vi "ConfigHelper.vi"(0 "object in":refnum<class "MTEC_Async.lvclass">, 2 "Config Data":T4={"meTEC_CH1_Input Selection (ID 2000)"=2, "meTEC_CH2_Input Selection (ID 2000)"=2, "meTEC_CH1_Object Target Temp. Source Selection (ID 50011)"=0, "meTEC_CH2_Object Target Temp. Source Selection (ID 50011)"=0, "meTEC_CH1_Live Enable (ID 50000)"=0, "meTEC_CH2_Live Enable (ID 50000)"=0, "meTEC_CH1_Object Target Temperature (ID 3000 / 50012) [°C]"=23.0, "meTEC_CH2_Object Target Temperature (ID 3000 / 50012) [°C]"=23.0, "meTEC_CH1_Live Set Current (ID 50001) [A]"=0.0, "meTEC_CH2_Live Set Current (ID 50001) [A]"=0.0, "meTEC_CH1_Live Set Voltage (ID 50002) [V]"=0.0, "meTEC_CH2_Live Set Voltage (ID 50002) [V]"=0.0} {"meTEC_CH2_Live Set Voltage (ID 50002) [V]" min=0.0 max=22.000001907348633 step=0.001 format="%#.3f"; "meTEC_CH1_Live Set Voltage (ID 50002) [V]" min=0.0 max=0.0 step=0.001 format="%#.3f"; "meTEC_CH2_Live Set Current (ID 50001) [A]" min=-10.0 max=10.0 step=0.001 format="%#.3f"; "meTEC_CH1_Live Set Current (ID 50001) [A]" min=0.0 max=0.0 step=0.001 format="%#.3f"; "meTEC_CH2_Object Target Temperature (ID 3000 / 50012) [°C]" min=-273.0 max=1000.0 step=0.001 format="%#.3f"; "meTEC_CH1_Object Target Temperature (ID 3000 / 50012) [°C]" min=0.0 max=0.0 step=0.001 format="%#.3f"; "meTEC_CH2_Live Enable (ID 50000)" items=["Disabled (Reset State)", "Enabled"]; "meTEC_CH1_Live Enable (ID 50000)" items=["Disabled (Reset State)", "Enabled"]; "meTEC_CH2_Object Target Temp. Source Selection (ID 50011)" items=["Parameter ID 3000 (Reset State)", "Parameter ID 50012"]; "meTEC_CH1_Object Target Temp. Source Selection (ID 50011)" items=["Parameter ID 3000 (Reset State)", "Parameter ID 50012"]; "meTEC_CH2_Input Selection (ID 2000)" items=["Static Current / Voltage", "Live Current / Voltage", "Temperature Controller"]; "meTEC_CH1_Input Selection (ID 2000)" items=["Static Current / Voltage", "Live Current / Voltage", "Temperature Controller"]}, 5 "error in (no error)":errorcluster) -> (14 "object out":refnum<class "MTEC_Async.lvclass">, 19 "error out":errorcluster)   [LabVIEW 2019, in "MTEC_Async.lvclass"]
uses:
  MTEC_Async.lvclass
  TEC LabVIEW Control Software v0.14/Source/LV Source/[meerstetter engineering TE Cooling]/TypeDefs/meTEC_ID 2000_Input Selection.ctl
  TEC LabVIEW Control Software v0.14/Source/LV Source/[meerstetter engineering TE Cooling]/TypeDefs/meTEC_ID 50011_Object Target Temperature Source Selection.ctl
  TEC LabVIEW Control Software v0.14/Source/LV Source/[meerstetter engineering TE Cooling]/TypeDefs/meTEC_ID 50000_Live Enable.ctl
  MTEC_Async.lvclass/MTEC_Async.ctl
  TEC LabVIEW Control Software v0.14/Source/LV Source/Variables/FGVs/Type Defs/FGV_Operations.ctl
panel:
  in  "meTEC_CH2_Live Set Voltage (ID 50002) [V]":dbl caption="Live Set Voltage (ID 50002) [V]" min=0.0 max=22.000001907348633 step=0.001 format="%#.3f"
  in  "meTEC_CH1_Live Set Voltage (ID 50002) [V]":dbl caption="Live Set Voltage (ID 50002) [V]" min=0.0 max=0.0 step=0.001 format="%#.3f"
  in  "meTEC_CH2_Live Set Current (ID 50001) [A]":dbl caption="Live Set Current (ID 50001) [A]" min=-10.0 max=10.0 step=0.001 format="%#.3f"
  in  "meTEC_CH1_Live Set Current (ID 50001) [A]":dbl caption="Live Set Current (ID 50001) [A]" min=0.0 max=0.0 step=0.001 format="%#.3f"
  in  "meTEC_CH2_Object Target Temperature (ID 3000 / 50012) [°C]":dbl
  in  "meTEC_CH1_Object Target Temperature (ID 3000 / 50012) [°C]":dbl=23.0 caption="Object Target Temperature (ID 3000 / 50012) [°C]" min=0.0 max=0.0 step=0.001 format="%#.3f"
  in  "meTEC_CH2_Live Enable (ID 50000)":T1 caption="Live Enable" items=["Disabled (Reset State)", "Enabled"]
  in  "meTEC_CH1_Live Enable (ID 50000)":T1 caption="Live Enable (ID 50000)" items=["Disabled (Reset State)", "Enabled"]
  in  "meTEC_CH2_Object Target Temp. Source Selection (ID 50011)":T2 caption="Object Target Temperature Source Selection (ID 50011)" items=["Parameter ID 3000 (Reset State)", "Parameter ID 50012"]
  in  "meTEC_CH1_Object Target Temp. Source Selection (ID 50011)":T2 caption="Object Target Temperature Source Selection (ID 50011)" items=["Parameter ID 3000 (Reset State)", "Parameter ID 50012"]
  in  "meTEC_CH2_Input Selection (ID 2000)":T3=2 caption="Input  Selection (ID 2000)" items=["Static Current / Voltage", "Live Current / Voltage", "Temperature Controller"]
  in  "meTEC_CH1_Input Selection (ID 2000)":T3=2 caption="Input  Selection (ID 2000)" items=["Static Current / Voltage", "Live Current / Voltage", "Temperature Controller"]
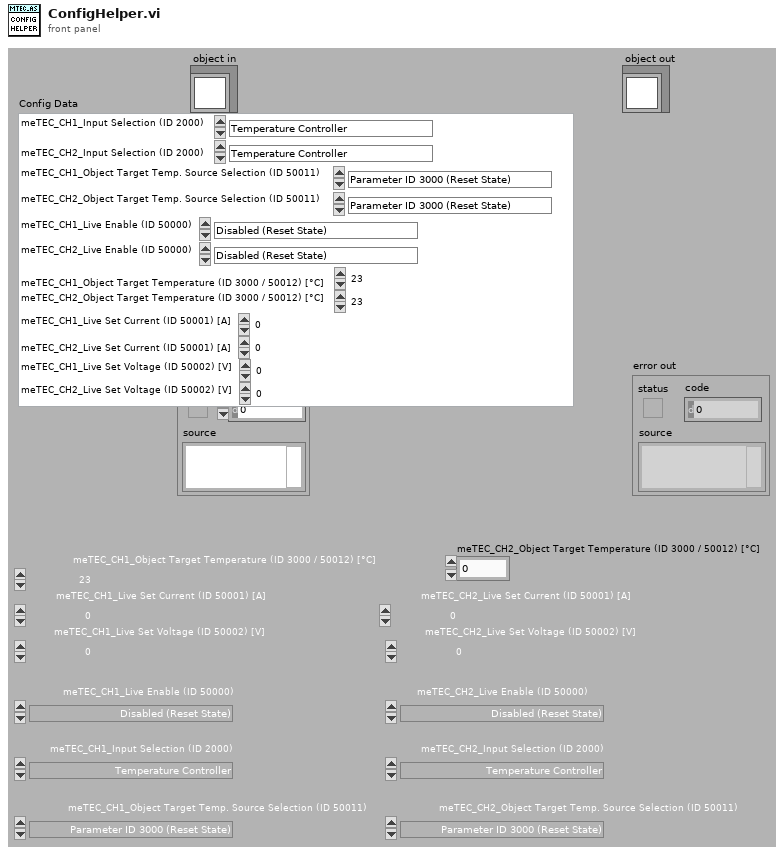
[diagram p1: front panel]
types:
  T1 = typedef "meTEC_ID 50000_Live Enable.ctl" = i32
  T2 = typedef "meTEC_ID 50011_Object Target Temperature Source Selection.ctl" = i32
  T3 = typedef "meTEC_ID 2000_Input Selection.ctl" = i32
  T4 = cluster{"meTEC_CH1_Input Selection (ID 2000)":T3, "meTEC_CH2_Input Selection (ID 2000)":T3, "meTEC_CH1_Object Target Temp. Source Selection (ID 50011)":T2, "meTEC_CH2_Object Target Temp. Source Selection (ID 50011)":T2, "meTEC_CH1_Live Enable (ID 50000)":T1, "meTEC_CH2_Live Enable (ID 50000)":T1, "meTEC_CH1_Object Target Temperature (ID 3000 / 50012) [°C]":dbl, "meTEC_CH2_Object Target Temperature (ID 3000 / 50012) [°C]":dbl, "meTEC_CH1_Live Set Current (ID 50001) [A]":dbl, "meTEC_CH2_Live Set Current (ID 50001) [A]":dbl, "meTEC_CH1_Live Set Voltage (ID 50002) [V]":dbl, "meTEC_CH2_Live Set Voltage (ID 50002) [V]":dbl}
  T5 = typedef "FGV_Operations.ctl" = enum16{"Read", "Write"}
  T6 = typedef "FGV_TE Controller.ctl" = cluster{"SVs":cluster{"Unused":dbl}, "PVs":cluster{"FW & HW Versions":cluster{"Device Type [I32]":i32, "Device Type [String]":string, "Firmware Version [I32]":i32, "Firmware Version [String]":string, "Hardware Version [I32]":i32, "Hardware Version [String]":string, "Serial No.":i32}, "TEC Configuration":T7, "Object Target Temperature Source_CH1":u8, "Object Target Temperature Source_CH2":u8}, "Front Panel References":T8}
  T7 = typedef "meTEC_Configuration.ctl" = cluster{"VISA resource name":refnum<visa-resource-name>, "Device Address":u16}
  T8 = typedef "FGV_Front Panel References.ctl" = cluster{"Main Loop Queue":refnum<queue>, "meTEC_Device Type":refnum<vi>, "meTEC_Serial No.":refnum<vi>, "meTEC_Hardware Version":refnum<vi>, "meTEC_Firmware Version":refnum<vi>, "meTEC_CH1_Object Target Temperature (ID 3000 / 50012) [°C]":refnum<vi>, "meTEC_CH1_Live Set Current (ID 50001) [A]":refnum<vi>, "meTEC_CH1_Live Set Voltage (ID 50002) [V]":refnum<vi>, "meTEC_CH1_Live Enable (ID 50000)":refnum<vi>, "meTEC_CH1_Input Selection (ID 2000)":refnum<vi>, "meTEC_CH1_Object Target Temp. Source Sel. (ID 50011)":refnum<vi>, "meTEC_CH2_Object Target Temperature (ID 3000 / 50012) [°C]":refnum<vi>, "meTEC_CH2_Live Set Current (ID 50001) [A]":refnum<vi>, "meTEC_CH2_Live Set Voltage (ID 50002) [V]":refnum<vi>, "meTEC_CH2_Live Enable (ID 50000)":refnum<vi>, "meTEC_CH2_Input Selection (ID 2000)":refnum<vi>, "meTEC_CH2_Object Target Temp. Source Sel. (ID 50011)":refnum<vi>, "meTEC_CH2_Object Temperature [°C]":refnum<vi>, "meTEC_CH2_Sink Temperature [°C]":refnum<vi>, "meTEC_CH2_Act. Output Current [A]":refnum<vi>, "meTEC_CH2_Act. Output Voltage [V]":refnum<vi>, "meTEC_CH2_Temperature Stability":refnum<vi>, "Monitor Chart_CH2":refnum<vi>, "meTEC_Initialize Device":refnum<vi>}
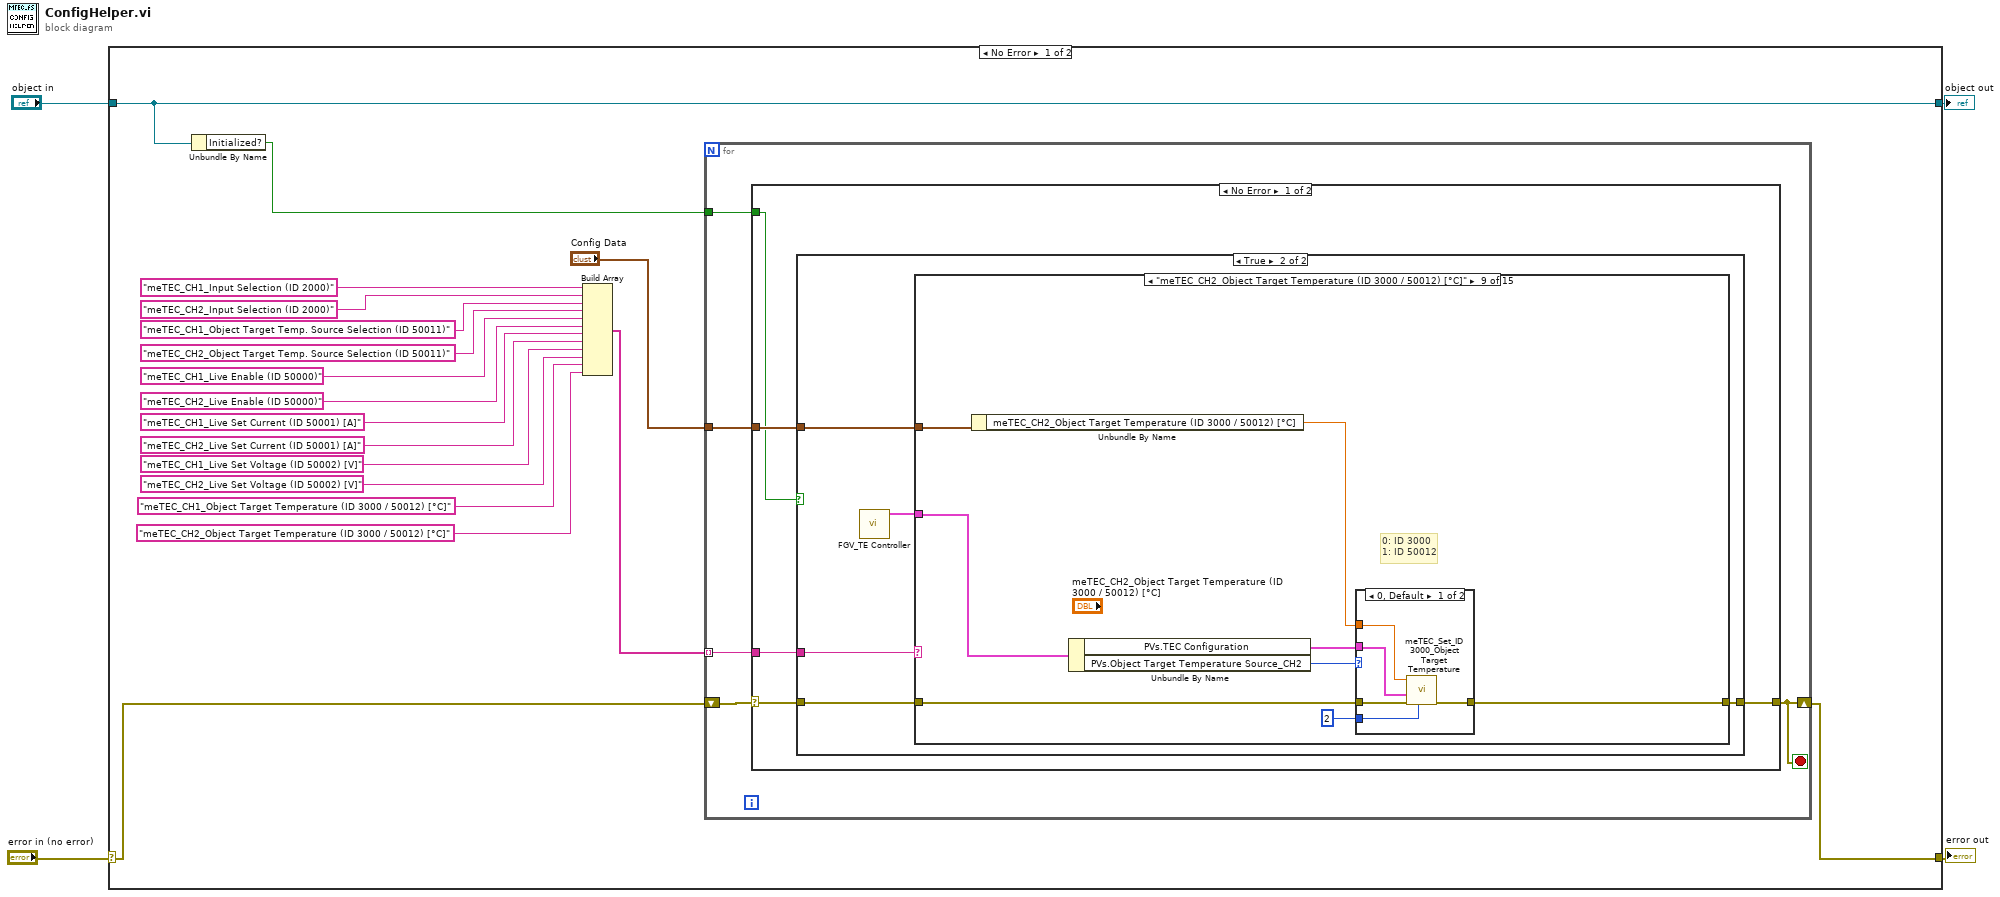
[diagram p0: block diagram]
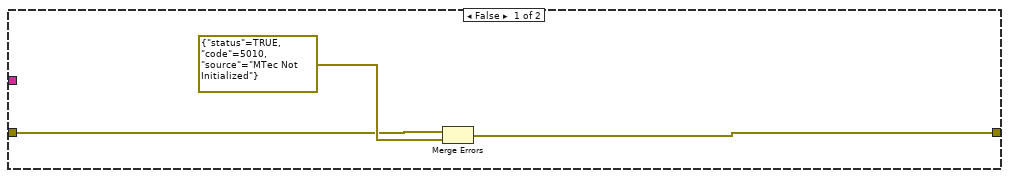
[diagram p2: hidden frame]
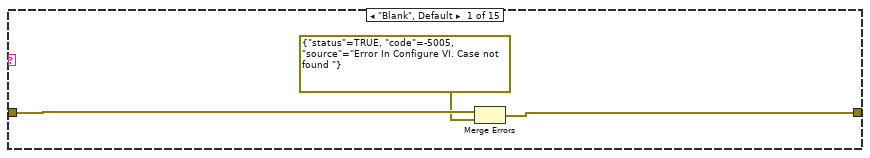
[diagram p3: hidden frame]
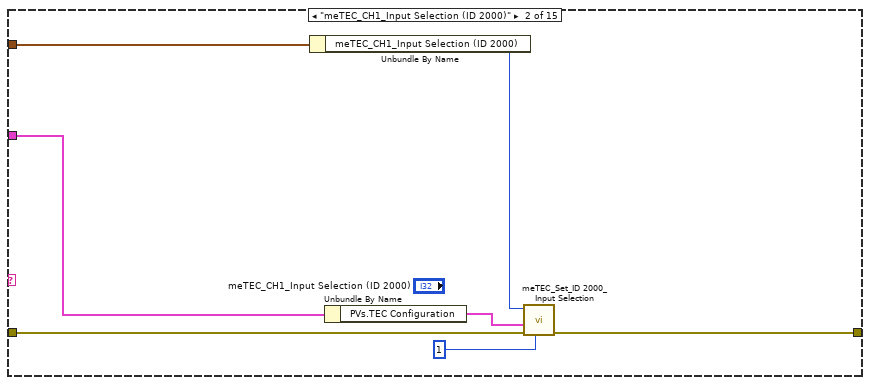
[diagram p4: hidden frame]
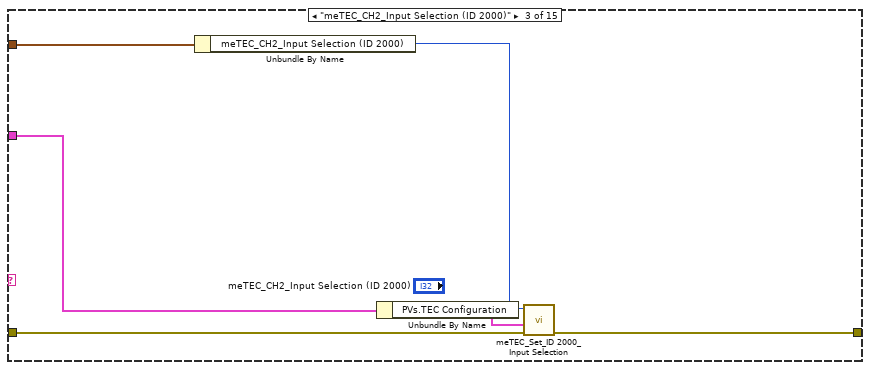
[diagram p5: hidden frame]
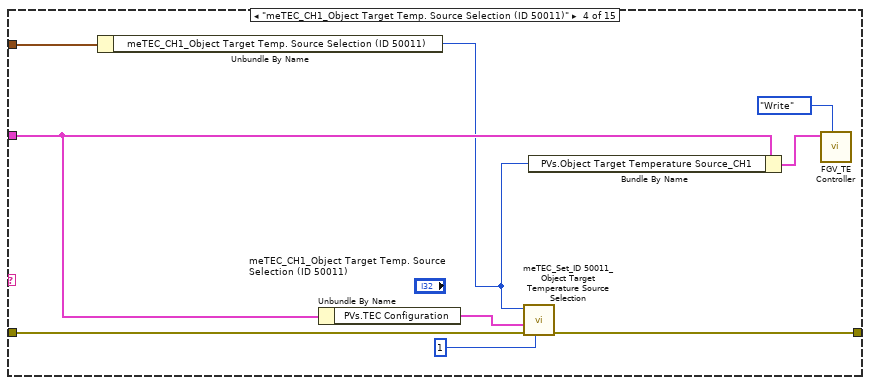
[diagram p6: hidden frame]
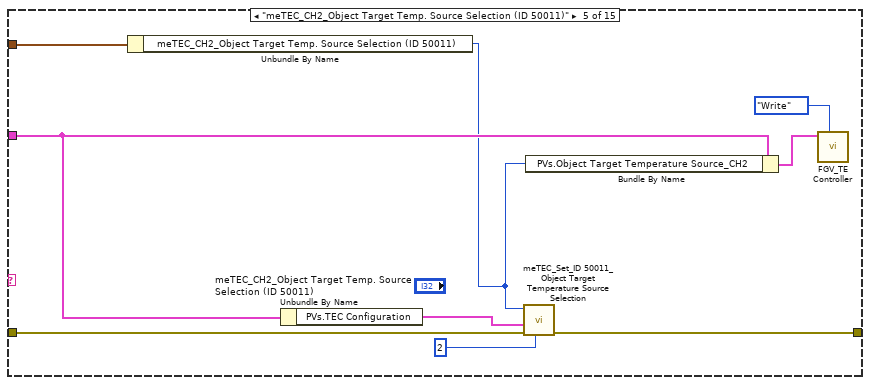
[diagram p7: hidden frame]
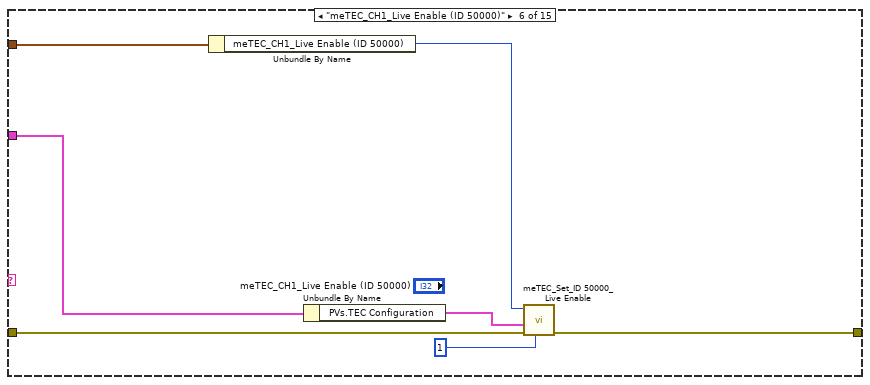
[diagram p8: hidden frame]
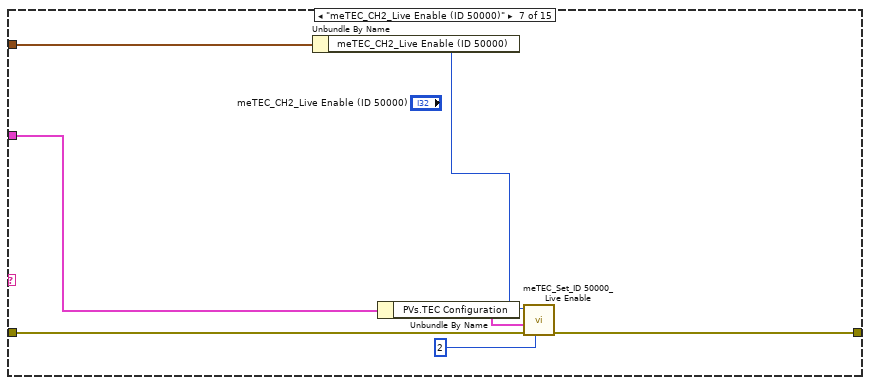
[diagram p9: hidden frame]
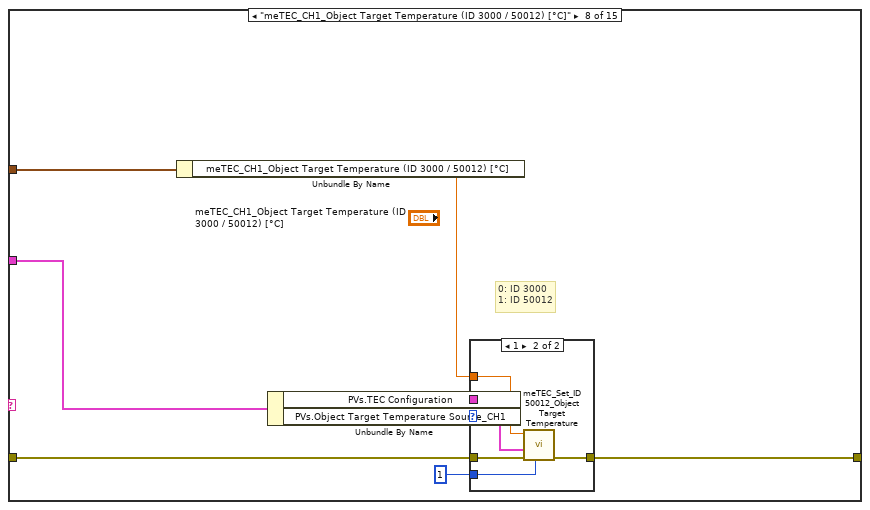
[diagram p10: hidden frame]
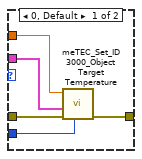
[diagram p11: hidden frame]
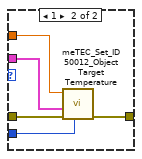
[diagram p12: hidden frame]
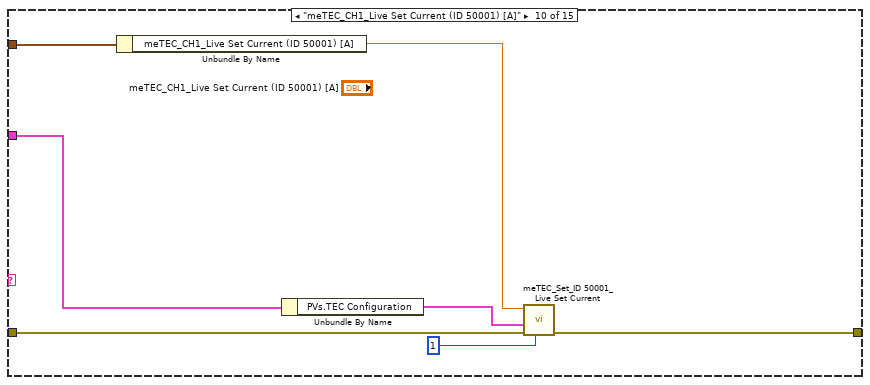
[diagram p13: hidden frame]
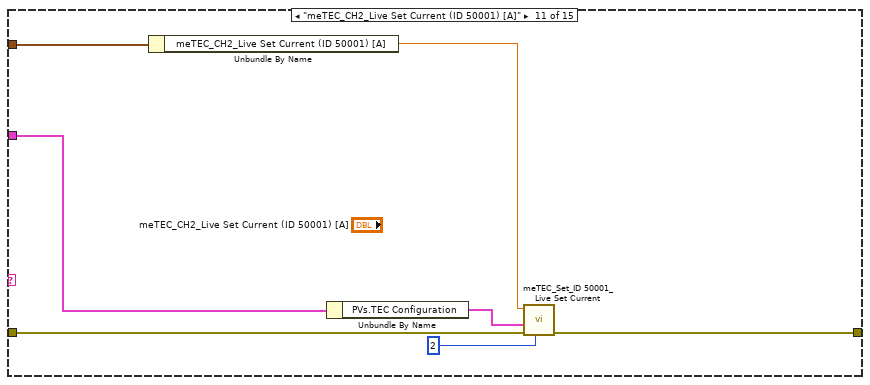
[diagram p14: hidden frame]
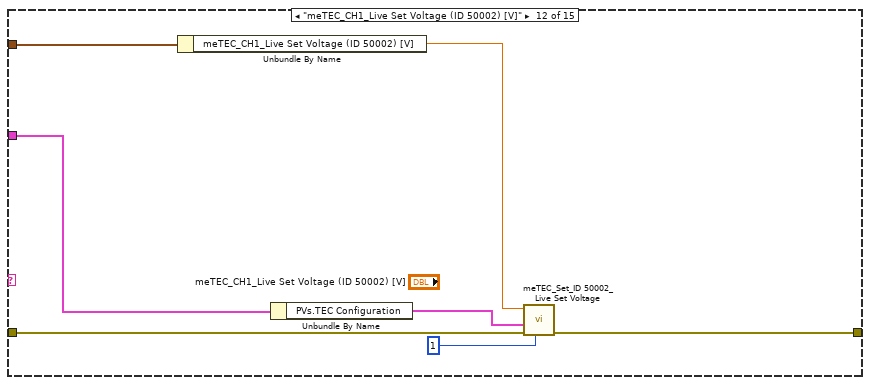
[diagram p15: hidden frame]
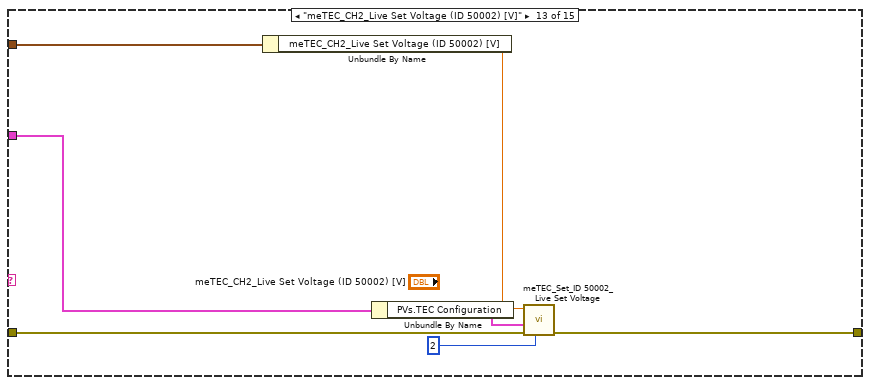
[diagram p16: hidden frame]
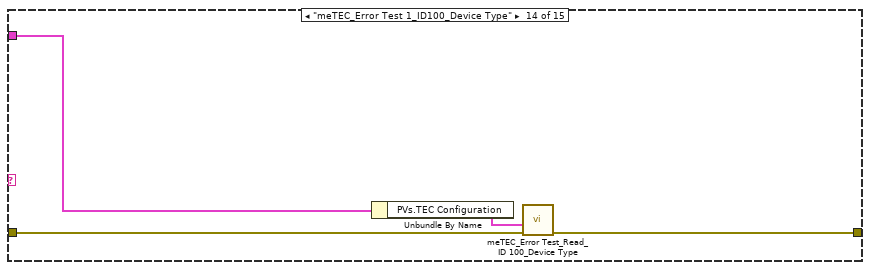
[diagram p17: hidden frame]
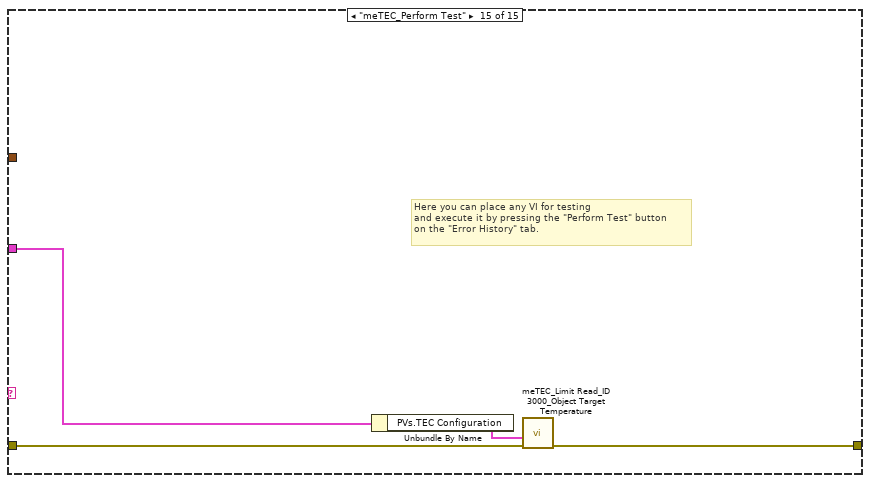
[diagram p18: hidden frame]
diagram:
  n1 = case shown="No Error" "error in (no error)" {
    selector: "error in (no error)" -> [w5 w163]
    tunnel: [w6 w163] -> w3
    tunnel: [w22 w162] -> w1
    tunnel: "object in" -> [w22 w162]
    frame No Error {
      n2 = Unbundle By Name(w22) -> ("Initialized?"=w7:bool)
      n3 = Build Array("meTEC_CH1_Input Selection (ID 2000)", "meTEC_CH2_Input Selection (ID 2000)", "meTEC_CH1_Object Target Temp. Source Selection (ID 50011)", "meTEC_CH2_Object Target Temp. Source Selection (ID 50011)", "meTEC_CH1_Live Enable (ID 50000)", "meTEC_CH2_Live Enable (ID 50000)", "meTEC_CH1_Live Set Current (ID 50001) [A]", "meTEC_CH2_Live Set Current (ID 50001) [A]", "meTEC_CH1_Live Set Voltage (ID 50002) [V]", "meTEC_CH2_Live Set Voltage (ID 50002) [V]", "meTEC_CH1_Object Target Temperature (ID 3000 / 50012) [°C]", "meTEC_CH2_Object Target Temperature (ID 3000 / 50012) [°C]") -> (w10:string[])
      n4 = for {
        tunnel: w10 -> [w26] mode=indexing
        tunnel: "Config Data" -> [w25]
        shift-right: [w23] -> w6
        shift-left: w5 -> [w27]
        tunnel: w7 -> [w24]
        stop <- w23 stop-if-true
        n5 = case shown="No Error" w27 {
          selector: w27 -> [w31 w161]
          tunnel: [w30 w161] -> w23
          tunnel: w26 -> [w32 _]
          tunnel: w25 -> [w29 _]
          tunnel: w24 -> [w28 _]
          frame No Error {
            n6 = case shown="True" w28 {
              tunnel: w32 -> [_ w39]
              tunnel: w31 -> [w33 w38]
              tunnel: [w34 w37] -> w30
              tunnel: w29 -> [_ w36]
              frame False {
                n7 = Merge Errors(w33, errorcluster {"status"=TRUE, "code"=5010, "source"="MTec Not Initialized"} ("error in (no error)")) -> (w34:errorcluster)
              }
              frame True {
                n8 = call "FGV_TE Controller.vi"() -> ("FGV_TEC_OUT"=w40:T6)  [unwired: 10 in, 1 out]
                n9 = case shown="\"meTEC_CH2_Object Target Temperature (ID 3000 / 50012) [°C]\"" w39 {
                  tunnel: w38 -> [w43 w50 w56 w65 w74 w81 w88 w96 w114 w131 w138 w145 w152 w155 w159]
                  tunnel: [w42 w49 w55 w64 w73 w80 w87 w95 w113 w130 w137 w144 w151 w153 w157] -> w37
                  tunnel: w40 -> [_ w48 w54 w61 w68 w79 w86 w94 w112 w129 w136 w143 w150 w156 w160]
                  tunnel: w36 -> [_ w45 w52 w58 w67 w76 w83 w90 w108 w126 w133 w140 w147 _ _]
                  frame "Blank", Default {
                    n10 = Merge Errors(w43, errorcluster {"status"=TRUE, "code"=-5005, "source"="Error In Configure VI. Case not found "} ("error in (no error)")) -> (w42:errorcluster)
                  }
                  frame "meTEC_CH1_Input Selection (ID 2000)" {
                    n11 = Unbundle By Name(w45) -> ("meTEC_CH1_Input Selection (ID 2000)"=w44:T3)
                    n12 = Unbundle By Name(w48) -> ("PVs.TEC Configuration"=w47:T7)
                    n13 = call "meTEC_Set_ID 2000_Input Selection.vi"("Instance (1)"=u8 1, "error in (no error)"=w50, "TEC Configuration_IN"=w47, "Input Selection (ID 2000)"=w44) -> ("error out"=w49:errorcluster)  [unwired: 5 in, 2 out]
                  }
                  frame "meTEC_CH2_Input Selection (ID 2000)" {
                    n14 = Unbundle By Name(w52) -> ("meTEC_CH2_Input Selection (ID 2000)"=w51:T3)
                    n15 = Unbundle By Name(w54) -> ("PVs.TEC Configuration"=w53:T7)
                    n16 = call "meTEC_Set_ID 2000_Input Selection.vi"("error in (no error)"=w56, "TEC Configuration_IN"=w53, "Input Selection (ID 2000)"=w51) -> ("error out"=w55:errorcluster)  [unwired: 6 in, 2 out]
                  }
                  frame "meTEC_CH1_Object Target Temp. Source Selection (ID 50011)" {
                    n17 = Unbundle By Name(w58) -> ("meTEC_CH1_Object Target Temp. Source Selection (ID 50011)"=w57:T2)
                    n18 = Unbundle By Name(w61) -> ("PVs.TEC Configuration"=w63:T7)
                    n19 = call "meTEC_Set_ID 50011_Object Target Temperature Source Selection.vi"("Instance (1)"=u8 1 ("Instance (0)"), "error in (no error)"=w65, "TEC Configuration_IN"=w63, "Object Target Temperature Source Selection (ID 50011)"=w57) -> ("error out"=w64:errorcluster)  [unwired: 5 in, 2 out]
                    n20 = Bundle By Name(cluster=w61, "PVs.Object Target Temperature Source_CH1"=w57) -> (w60:T6)
                    n21 = call "FGV_TE Controller.vi"("Operation (Read)"=FGV_Operations."Write", "FGV_TEC_IN"=w60) -> ()  [unwired: 8 in, 2 out]
                  }
                  frame "meTEC_CH2_Object Target Temp. Source Selection (ID 50011)" {
                    n22 = Unbundle By Name(w67) -> ("meTEC_CH2_Object Target Temp. Source Selection (ID 50011)"=w66:T2)
                    n23 = Unbundle By Name(w68) -> ("PVs.TEC Configuration"=w72:T7)
                    n24 = call "meTEC_Set_ID 50011_Object Target Temperature Source Selection.vi"("Instance (1)"=u8 2 ("Instance (0)"), "error in (no error)"=w74, "TEC Configuration_IN"=w72, "Object Target Temperature Source Selection (ID 50011)"=w66) -> ("error out"=w73:errorcluster)  [unwired: 5 in, 2 out]
                    n25 = Bundle By Name(cluster=w68, "PVs.Object Target Temperature Source_CH2"=w66) -> (w69:T6)
                    n26 = call "FGV_TE Controller.vi"("Operation (Read)"=FGV_Operations."Write", "FGV_TEC_IN"=w69) -> ()  [unwired: 8 in, 2 out]
                  }
                  frame "meTEC_CH1_Live Enable (ID 50000)" {
                    n27 = Unbundle By Name(w76) -> ("meTEC_CH1_Live Enable (ID 50000)"=w75:T1)
                    n28 = Unbundle By Name(w79) -> ("PVs.TEC Configuration"=w78:T7)
                    n29 = call "meTEC_Set_ID 50000_Live Enable.vi"("Instance (1)"=u8 1 ("Instance (0)"), "error in (no error)"=w81, "TEC Configuration_IN"=w78, "Live Enable (ID 50000)"=w75) -> ("error out"=w80:errorcluster)  [unwired: 5 in, 2 out]
                  }
                  frame "meTEC_CH2_Live Enable (ID 50000)" {
                    n30 = Unbundle By Name(w83) -> ("meTEC_CH2_Live Enable (ID 50000)"=w82:T1)
                    n31 = Unbundle By Name(w86) -> ("PVs.TEC Configuration"=w85:T7)
                    n32 = call "meTEC_Set_ID 50000_Live Enable.vi"("Instance (1)"=u8 2 ("Instance (0)"), "error in (no error)"=w88, "TEC Configuration_IN"=w85, "Live Enable (ID 50000)"=w82) -> ("error out"=w87:errorcluster)  [unwired: 5 in, 2 out]
                  }
                  frame "meTEC_CH1_Object Target Temperature (ID 3000 / 50012) [°C]" {
                    # "0: ID 3000\n1: ID 50012"
                    n33 = Unbundle By Name(w90) -> ("meTEC_CH1_Object Target Temperature (ID 3000 / 50012) [°C]"=w89:dbl)
                    n34 = Unbundle By Name(w94) -> ("PVs.TEC Configuration"=w93:T7, "PVs.Object Target Temperature Source_CH1"=w91:u8)
                    n35 = case shown="1" w91 {
                      tunnel: w96 -> [w101 w106]
                      tunnel: [w100 w105] -> w95
                      tunnel: w89 -> [w99 w104]
                      tunnel: w93 -> [w98 w103]
                      tunnel: u8 1 ("Instance") -> [w97 w102]
                      frame 0, Default {
                        n36 = call "meTEC_Set_ID 3000_Object Target Temperature.vi"("Instance (1)"=w97, "error in (no error)"=w101, "TEC Configuration_IN"=w98, "Object Target Temperature [°C]"=w99) -> ("error out"=w100:errorcluster)  [unwired: 5 in, 2 out]
                      }
                      frame 1 {
                        n37 = call "meTEC_Set_ID 50012_Object Target Temperature.vi"("Instance (1)"=w102, "error in (no error)"=w106, "TEC Configuration_IN"=w103, "Object Target Temperature [°C]"=w104) -> ("error out"=w105:errorcluster)  [unwired: 5 in, 2 out]
                      }
                    }
                  }
                  frame "meTEC_CH2_Object Target Temperature (ID 3000 / 50012) [°C]" {
                    # "0: ID 3000\n1: ID 50012"
                    n38 = Unbundle By Name(w108) -> ("meTEC_CH2_Object Target Temperature (ID 3000 / 50012) [°C]"=w107:dbl)
                    n39 = Unbundle By Name(w112) -> ("PVs.TEC Configuration"=w111:T7, "PVs.Object Target Temperature Source_CH2"=w109:u8)
                    n40 = case shown="0, Default" w109 {
                      tunnel: w114 -> [w119 w124]
                      tunnel: [w118 w123] -> w113
                      tunnel: w107 -> [w117 w122]
                      tunnel: w111 -> [w116 w121]
                      tunnel: u8 2 ("Instance") -> [w115 w120]
                      frame 0, Default {
                        n41 = call "meTEC_Set_ID 3000_Object Target Temperature.vi"("Instance (1)"=w115, "error in (no error)"=w119, "TEC Configuration_IN"=w116, "Object Target Temperature [°C]"=w117) -> ("error out"=w118:errorcluster)  [unwired: 5 in, 2 out]
                      }
                      frame 1 {
                        n42 = call "meTEC_Set_ID 50012_Object Target Temperature.vi"("Instance (1)"=w120, "error in (no error)"=w124, "TEC Configuration_IN"=w121, "Object Target Temperature [°C]"=w122) -> ("error out"=w123:errorcluster)  [unwired: 5 in, 2 out]
                      }
                    }
                  }
                  frame "meTEC_CH1_Live Set Current (ID 50001) [A]" {
                    n43 = Unbundle By Name(w126) -> ("meTEC_CH1_Live Set Current (ID 50001) [A]"=w125:dbl)
                    n44 = Unbundle By Name(w129) -> ("PVs.TEC Configuration"=w128:T7)
                    n45 = call "meTEC_Set_ID 50001_Live Set Current.vi"("Instance (1)"=u8 1 ("Instance"), "error in (no error)"=w131, "TEC Configuration_IN"=w128, "Live Current [A]"=w125) -> ("error out"=w130:errorcluster)  [unwired: 5 in, 2 out]
                  }
                  frame "meTEC_CH2_Live Set Current (ID 50001) [A]" {
                    n46 = Unbundle By Name(w133) -> ("meTEC_CH2_Live Set Current (ID 50001) [A]"=w132:dbl)
                    n47 = Unbundle By Name(w136) -> ("PVs.TEC Configuration"=w135:T7)
                    n48 = call "meTEC_Set_ID 50001_Live Set Current.vi"("Instance (1)"=u8 2 ("Instance"), "error in (no error)"=w138, "TEC Configuration_IN"=w135, "Live Current [A]"=w132) -> ("error out"=w137:errorcluster)  [unwired: 5 in, 2 out]
                  }
                  frame "meTEC_CH1_Live Set Voltage (ID 50002) [V]" {
                    n49 = Unbundle By Name(w140) -> ("meTEC_CH1_Live Set Voltage (ID 50002) [V]"=w139:dbl)
                    n50 = Unbundle By Name(w143) -> ("PVs.TEC Configuration"=w142:T7)
                    n51 = call "meTEC_Set_ID 50002_Live Set Voltage.vi"("Instance (1)"=u8 1 ("Instance"), "error in (no error)"=w145, "TEC Configuration_IN"=w142, "Live Set Voltage [V]"=w139) -> ("error out"=w144:errorcluster)  [unwired: 5 in, 2 out]
                  }
                  frame "meTEC_CH2_Live Set Voltage (ID 50002) [V]" {
                    n52 = Unbundle By Name(w147) -> ("meTEC_CH2_Live Set Voltage (ID 50002) [V]"=w146:dbl)
                    n53 = Unbundle By Name(w150) -> ("PVs.TEC Configuration"=w149:T7)
                    n54 = call "meTEC_Set_ID 50002_Live Set Voltage.vi"("Instance (1)"=u8 2 ("Instance"), "error in (no error)"=w152, "TEC Configuration_IN"=w149, "Live Set Voltage [V]"=w146) -> ("error out"=w151:errorcluster)  [unwired: 5 in, 2 out]
                  }
                  frame "meTEC_Error Test 1_ID100_Device Type" {
                    n55 = Unbundle By Name(w156) -> ("PVs.TEC Configuration"=w154:T7)
                    n56 = call "meTEC_Error Test_Read_ID 100_Device Type.vi"("error in (no error)"=w155, "TEC Configuration_IN"=w154) -> ("error out"=w153:errorcluster)  [unwired: 6 in, 3 out]
                  }
                  frame "meTEC_Perform Test" {
                    # "Here you can place any VI for testing \nand execute it by pressing the \"Perform Test\" button\non the \"Error History\" tab."
                    n57 = Unbundle By Name(w160) -> ("PVs.TEC Configuration"=w158:T7)
                    n58 = call "meTEC_Limit Read_ID 3000_Object Target Temperature.vi"("error in (no error)"=w159, "TEC Configuration_IN"=w158) -> ("error out"=w157:errorcluster)  [unwired: 6 in, 3 out]
                  }
                }
              }
            }
          }
          frame Error {
          }
        }
      }
    }
    frame Error {
    }
  }
  "error out" <- w3
  "object out" <- w1
